vi "Add heather.vi"(9 "value":string, 11 "header":string) -> (2 "headers":T1[](array[typedef]))   [LabVIEW 2021]
uses:
  <vilib>/addons/_JKI.lib/REST Client/classes/REST Client/HTTP Header.ctl
  <vilib>/addons/_JKI.lib/REST Client/classes/REST Client/REST Client.lvclass
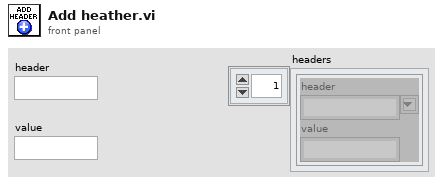
[diagram p1: front panel]
types:
  T1 = typedef "REST Client.lvlib/REST Client.lvclass/HTTP Header.ctl" = cluster{"header":string, "value":string}
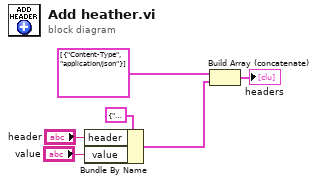
[diagram p0: block diagram]
diagram:
  n1 = Bundle By Name(cluster=cluster{"header":string, "value":string} {"header"="", "value"=""}, "header"="header", "value"="value") -> (w4:cluster{"header":string, "value":string})
  n2 = Build Array (concatenate)(T1[] [{"header"="Content-Type", "value"="application/json"}] ("Default Headers ([JSON])"), w4) -> (→"headers":T1[])
